vi "Angle between two vectors.vi"(10 "Vector 2":dbl[](array[numeric]), 11 "Vector 1":dbl[](array[numeric])) -> (1 "Angle (Degrees)":dbl, 2 "Angle (Radians)":dbl, 3 "Cos (Theta)":dbl)   [LabVIEW 2010]
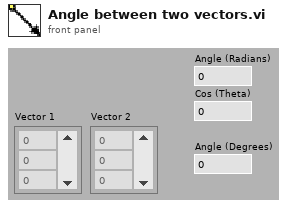
[diagram p1: front panel]
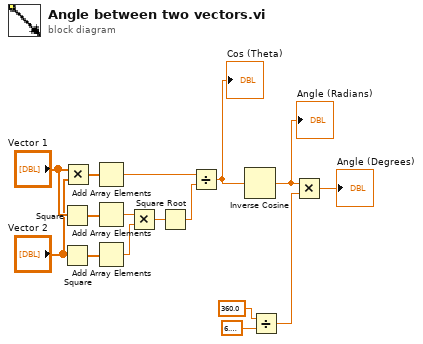
[diagram p0: block diagram]
diagram:
  n1 = Square(x="Vector 1") -> (x^2=w15:dbl[])
  n2 = Square(x="Vector 2") -> (x^2=w16:dbl[])
  n3 = Multiply(x="Vector 1", y="Vector 2") -> (x*y=w5:dbl[])
  n4 = Add Array Elements(numeric array=w5) -> (sum=w14:dbl)
  n5 = Add Array Elements(numeric array=w15) -> (sum=w4:dbl)
  n6 = Add Array Elements(numeric array=w16) -> (sum=w3:dbl)
  n7 = Multiply(x=w4, y=w3) -> (x*y=w2:dbl)
  n8 = Square Root(x=w2) -> (sqrt(x)=w1:dbl)
  n9 = Divide(x=w14, y=w1) -> (x/y=w13:dbl)
  "Cos (Theta)" <- w13
  n10 = Inverse Cosine(1:w13) -> (0:w9:dbl)
  "Angle (Radians)" <- w9
  n11 = Divide(x=360.0, y=6.283185307179586) -> (x/y=w10:dbl)
  n12 = Multiply(x=w9, y=w10) -> (x*y=→"Angle (Degrees)":dbl)
